vi "GxSingleCam.vi"() -> ()   [LabVIEW 2013]
uses:
  C:/Program Files/Daheng Imaging/GalaxySDK/Samples/LabVIEW SDK/x86/GxLVLib/dll/GxIAPINET.dll
  GxLVLib/dll/GxIAPINET.dll
  <vilib>/vision/Image Controls.llb/IMAQ Image.ctl
  GxLVLib/GxLVlib.lvlib
panel:
  out "是否退出":bool
  in  "图片存储路径":path
  in  "保存图片":bool
  in  "Image Src":T1
  out "Image":T1(plugin-control)
  out "采集回调":refnum<k27>
  out "是否支持白平衡":bool
  out "采集状态":bool
  out "设备状态":bool
  in  "IGxFactory":refnum<k24>
  in  "安全退出":bool
  in  "IGxStream":refnum<k24>
  in  "IGxDevice":refnum<k24>
  out "error out":errorcluster
  in  "发送软触发":bool
  in  "自动白平衡":string(combo)
  in  "增益":dbl format="%#_6f"
  in  "曝光时间":dbl
  in  "触发源":string(combo)
  in  "触发模式":string(combo)
  in  "停止采集":bool
  in  "开始采集":bool
  in  "关闭设备":bool
  in  "打开设备":bool
  # "触发模式"
  # "触发源"
  # "软触发"
  # "曝光时间(us)"
  # "增益(dB)"
  # "自动白平衡"
  # "保存图片"
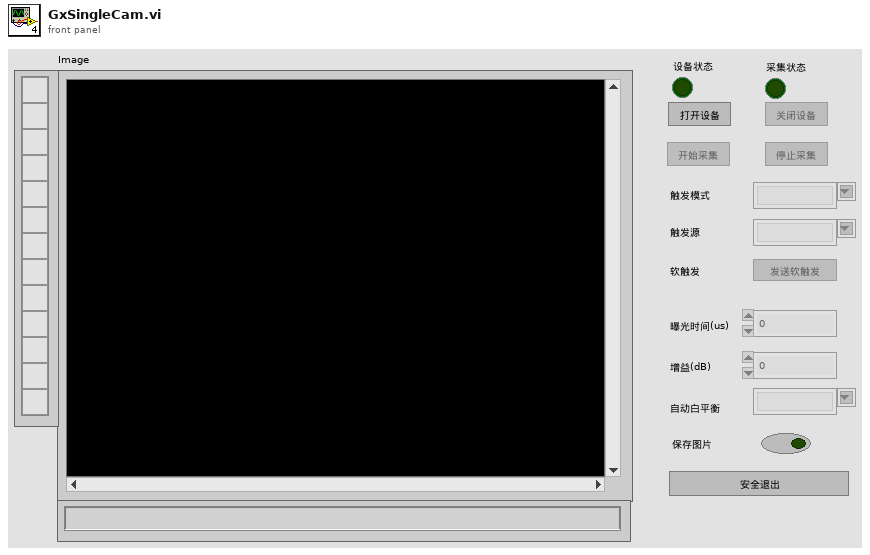
[diagram p1: front panel]
types:
  T1 = typedef "IMAQ Image.ctl" = refnum<image>
  T2 = typedef "Semaphore RefNum" = refnum<k1>
  T3 = enum8{"Enabled", "Disabled", "Disabled and Grayed Out"}
  T4 = typedef "Image Type" = u32
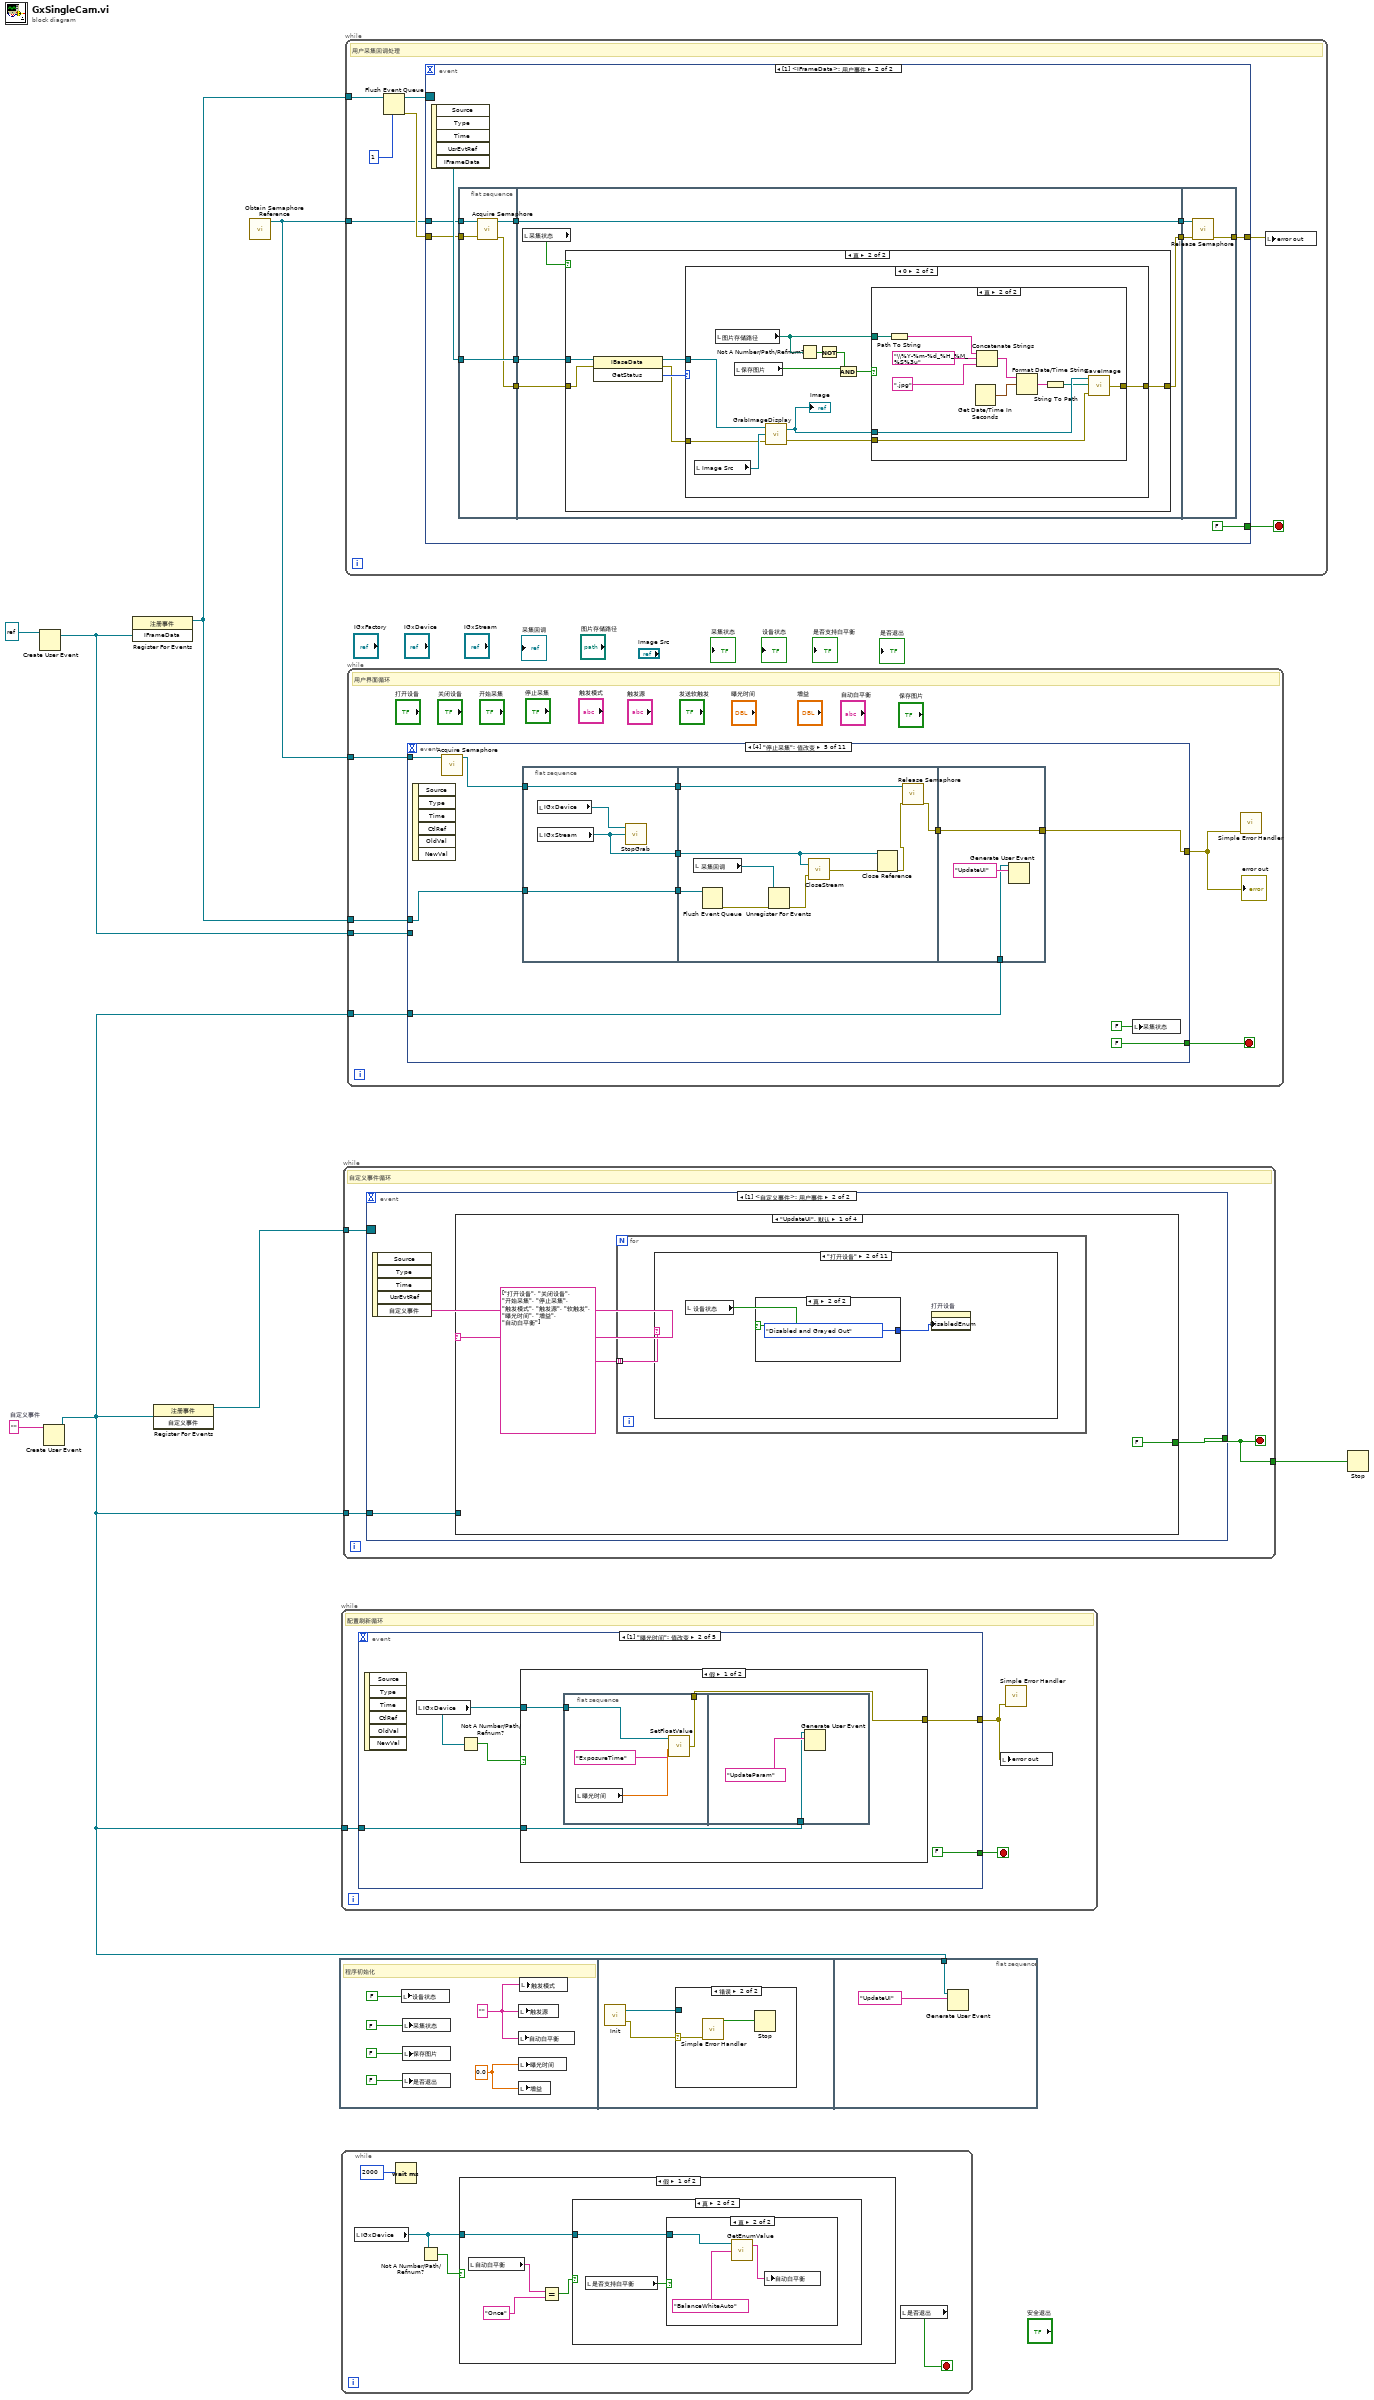
[diagram p0: block diagram]
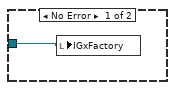
[diagram p5: hidden frame]
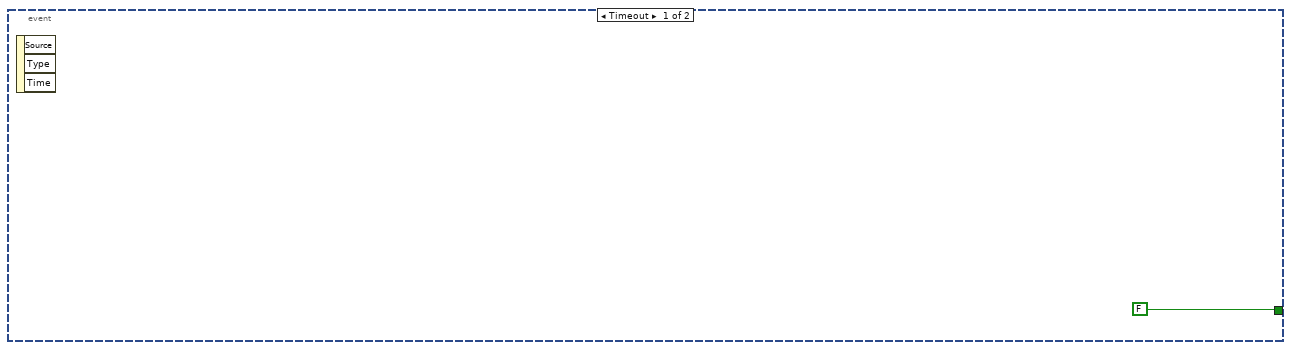
[diagram p6: hidden frame]
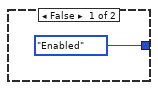
[diagram p8: hidden frame]
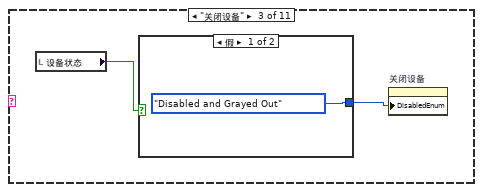
[diagram p9: hidden frame]
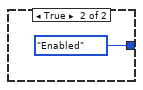
[diagram p10: hidden frame]
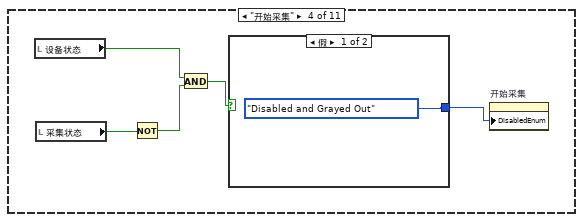
[diagram p11: hidden frame]
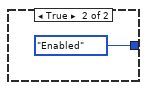
[diagram p12: hidden frame]
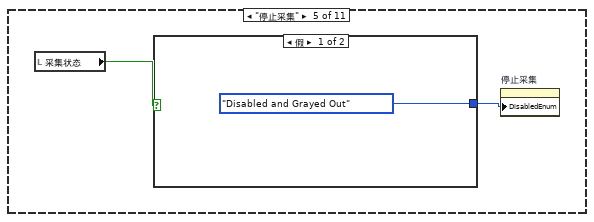
[diagram p13: hidden frame]
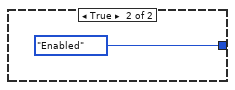
[diagram p14: hidden frame]
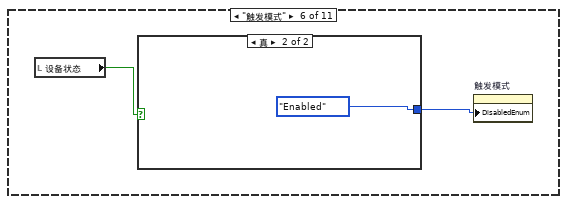
[diagram p15: hidden frame]
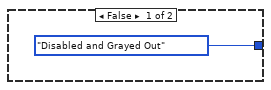
[diagram p16: hidden frame]
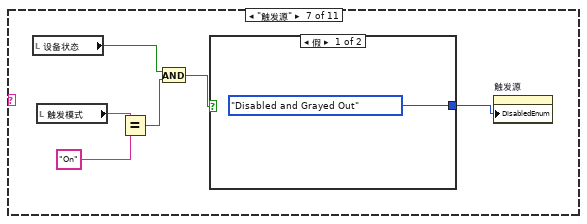
[diagram p17: hidden frame]
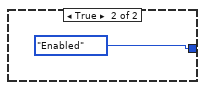
[diagram p18: hidden frame]
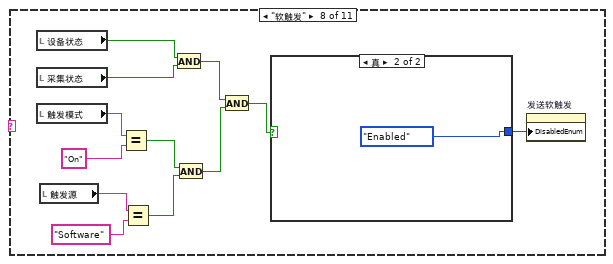
[diagram p19: hidden frame]
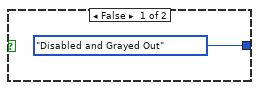
[diagram p20: hidden frame]
diagram:
  w6 = ""  # 自定义事件
  n1 = Create User Event(user event datatype=refnum<k24> refnum ("IFrameData")) -> (user event=w8:refnum<user-event>)  [unwired: 1 in, 1 out]
  n2 = Create User Event(user event datatype=w6) -> (user event=w3:refnum<user-event>)  [unwired: 1 in, 1 out]
  n3 = register-events(w8) -> (reference out=w2:refnum<event-registration>)  [unwired: 2 in, 1 out]
  n4 = register-events(w3) -> (reference out=w5:refnum<event-registration>)  [unwired: 2 in, 1 out]
  n5 = call <vilib>:"Obtain Semaphore Reference.vi"() -> ("semaphore"=w1:T2)  [unwired: 5 in, 2 out]
  n6 = flat-sequence {
    tunnel: w3 -> [w20]
    frame #0 {
      w11 = 0.0
      w12 = ""
      # "程序初始化"
      n7 = local write "设备状态"(FALSE) -> ()
      n8 = local write "采集状态"(FALSE) -> ()
      n9 = local write "保存图片"(FALSE) -> ()
      n10 = local write "是否退出"(FALSE) -> ()
      n11 = local write "自动白平衡"(w12) -> ()
      n12 = local write "触发源"(w12) -> ()
      n13 = local write "曝光时间"(w11) -> ()
      n14 = local write "增益"(w11) -> ()
      n15 = local write "触发模式"(w12) -> ()
    }
    frame #1 {
      n16 = call "Init.vi"() -> ("IGxFactory"=w16:refnum<k24>, "error out"=w15:errorcluster)  [unwired: 1 in]
      n17 = case shown="错误" w15 {
        selector: w15 -> [_ w18]
        tunnel: w16 -> [w17 _]
        frame No Error {
          n18 = local write "IGxFactory"(w17) -> ()
        }
        frame Error {
          n19 = call <vilib>:"Simple Error Handler.vi"("error in (no error)"=w18) -> ("error?"=w19:bool)  [unwired: 4 in, 4 out]
          n20 = Stop(stop? (T)=w19) -> ()
        }
      }
    }
    frame #2 {
      n21 = Generate User Event(user event=w20, event data cluster="UpdateUI") -> ()  [unwired: 2 in, 2 out]
    }
  }
  n22 = while {
    tunnel: w3 -> [w22]
    stop <- w24 stop-if-true
    # "配置刷新循环"
    n23 = event shown="[1] \"曝光时间\": 值改变" {
      selector: _ -> [_ _ _ _ _]
      dyn-events: _ -> [_ _ _ _ _]
      timeout: _ -> [_ _ _ _ _]
      tunnel: [errorcluster {FALSE, 0, ""} w29 w44 w59 errorcluster {"status"=FALSE, "code"=0, "source"=""} ("错误常量")] -> w23
      tunnel: [FALSE FALSE FALSE FALSE TRUE] -> w24
      tunnel: w22 -> [_ w27 w42 w57 _]
      event Timeout {
        n24 = event-data() -> ()  [unwired: 1 in, 3 out]
      }
      event "曝光时间": Value Change {
        n25 = event-data() -> ()  [unwired: 1 in, 6 out]
        n26 = local read "IGxDevice"() -> (w30:refnum<k24>)
        n27 = Not A Number/Path/Refnum?(number/path/refnum=w30) -> (NaN/Path/Refnum?=w31:bool)
        n28 = case shown="假" w31 {
          tunnel: w30 -> [w34 _]
          tunnel: [w33 errorcluster {TRUE, 5000, "GxSingleCam.vi"}] -> w29
          tunnel: w27 -> [w32 _]
          frame False {
            n29 = flat-sequence {
              tunnel: w34 -> [w36]
              tunnel: [w35] -> w33
              tunnel: w32 -> [w39]
              frame #0 {
                n30 = local read "曝光时间"() -> (w38:dbl)
                n31 = call "SetFloatValue.vi"("Float Value"=w38, "Feature Name"="ExposureTime", "IGxDevice"=w36) -> ("error out"=w35:errorcluster)  [unwired: 1 in]
              }
              frame #1 {
                n32 = Generate User Event(user event=w39, event data cluster="UpdateParam") -> ()  [unwired: 2 in, 2 out]
              }
            }
          }
          frame True {
          }
        }
      }
      event "增益": Value Change {
        n33 = event-data() -> ()  [unwired: 1 in, 6 out]
        n34 = local read "IGxDevice"() -> (w46:refnum<k24>)
        n35 = Not A Number/Path/Refnum?(number/path/refnum=w46) -> (NaN/Path/Refnum?=w45:bool)
        n36 = case shown="真" w45 {
          tunnel: w46 -> [w49 _]
          tunnel: [w48 errorcluster {TRUE, 0, "设备句柄无效"}] -> w44
          tunnel: w42 -> [w47 _]
          frame False {
            n37 = flat-sequence {
              tunnel: w49 -> [w51]
              tunnel: [w50] -> w48
              tunnel: w47 -> [w55]
              frame #0 {
                n38 = local read "增益"() -> (w53:dbl)
                n39 = call "SetFloatValue.vi"("Float Value"=w53, "Feature Name"="Gain", "IGxDevice"=w51) -> ("error out"=w50:errorcluster)  [unwired: 1 in]
              }
              frame #1 {
                n40 = Generate User Event(user event=w55, event data cluster="UpdateParam") -> ()  [unwired: 2 in, 2 out]
              }
            }
          }
          frame True {
          }
        }
      }
      event "自动白平衡": Value Change {
        n41 = event-data() -> ()  [unwired: 1 in, 6 out]
        n42 = local read "IGxDevice"() -> (w60:refnum<k24>)
        n43 = Not A Number/Path/Refnum?(number/path/refnum=w60) -> (NaN/Path/Refnum?=w61:bool)
        n44 = case shown="假" w61 {
          tunnel: w60 -> [w64 _]
          tunnel: [w63 errorcluster {TRUE, 0, "设备句柄无效"}] -> w59
          tunnel: w57 -> [w62 _]
          frame False {
            n45 = flat-sequence {
              tunnel: w64 -> [w66]
              tunnel: [w65] -> w63
              tunnel: w62 -> [w69]
              frame #0 {
                n46 = local read "自动白平衡"() -> (w68:string)
                n47 = call "SetEnumValue.vi"("Enum Value"=w68, "Feature Name"="BalanceWhiteAuto", "IGxDevice"=w66) -> ("error out"=w65:errorcluster)  [unwired: 1 in]
              }
              frame #1 {
                n48 = Generate User Event(user event=w69, event data cluster="UpdateParam") -> ()  [unwired: 2 in, 2 out]
              }
            }
          }
          frame True {
          }
        }
      }
      event "安全退出": Value Change {
        n49 = event-data() -> ()  [unwired: 1 in, 6 out]
      }
    }
    n50 = local write "error out"(w23) -> ()
    n51 = call <vilib>:"Simple Error Handler.vi"("error in (no error)"=w23) -> ()  [unwired: 4 in, 5 out]
  }
  n52 = while {
    stop <- w74 stop-if-true
    n53 = local read "IGxDevice"() -> (w76:refnum<k24>)
    n54 = Wait (ms)(milliseconds to wait=2000) -> ()  [unwired: 1 out]
    n55 = Not A Number/Path/Refnum?(number/path/refnum=w76) -> (NaN/Path/Refnum?=w75:bool)
    n56 = case shown="假" w75 {
      tunnel: w76 -> [w81 _]
      frame False {
        n57 = local read "自动白平衡"() -> (w79:string)
        n58 = Equal?(x=w79, y="Once") -> (x = y?=w78:bool)
        n59 = case shown="真" w78 {
          tunnel: w81 -> [_ w82]
          frame False {
          }
          frame True {
            n60 = local read "是否支持白平衡"() -> (w83:bool)
            n61 = case shown="真" w83 {
              tunnel: w82 -> [_ w86]
              frame False {
              }
              frame True {
                n62 = call "GetEnumValue.vi"("Feature Name"="BalanceWhiteAuto", "IGxDevice"=w86) -> ("Enum Value"=w84:string)  [unwired: 1 in, 1 out]
                n63 = local write "自动白平衡"(w84) -> ()
              }
            }
          }
        }
      }
      frame True {
      }
    }
    n64 = local read "是否退出"() -> (w74:bool)
  }
  n65 = while {
    tunnel: w5 -> [w89]
    tunnel: w3 -> [w88]
    tunnel: [w87] -> w4
    stop <- w87 stop-if-true
    # "自定义事件循环"
    n66 = event shown="[1] <自定义事件>: 用户事件" {
      selector: w89 -> [_ _]
      dyn-events: _ -> [_ _]
      timeout: _ -> [_ _]
      tunnel: [FALSE w91] -> w87
      tunnel: w88 -> [_ w92]
      event Timeout {
        n67 = event-data() -> ()  [unwired: 1 in, 3 out]
      }
      event User Event {
        n68 = event-data() -> ("自定义事件"=w93:string)  [unwired: 1 in, 4 out]
        n69 = case shown="\"UpdateUI\", 默认" w93 {
          tunnel: w92 -> [_ _ w224 _]
          tunnel: [FALSE TRUE FALSE FALSE] -> w91
          frame "UpdateUI", Default {
            n70 = for {
              tunnel: string[] ["打开设备", "关闭设备", "开始采集", "停止采集", "触发模式", "触发源", "软触发", "曝光时间", "增益", "自动白平衡"] -> [w96] mode=indexing
              n71 = case shown="\"打开设备\"" w96 {
                frame Default {
                }
                frame "打开设备" {
                  n72 = local read "设备状态"() -> (w98:bool)
                  n73 = case shown="真" w98 {
                    tunnel: [T3."Enabled" ("禁用") T3."Disabled and Grayed Out" ("禁用")] -> w97
                    frame False {
                    }
                    frame True {
                    }
                  }
                  n74 = property on="打开设备" class="Bool"("DisabledEnum"=w97) -> ()  [unwired: 2 in, 2 out]
                }
                frame "关闭设备" {
                  n75 = local read "设备状态"() -> (w102:bool)
                  n76 = case shown="假" w102 {
                    tunnel: [T3."Disabled and Grayed Out" ("禁用") T3."Enabled" ("禁用")] -> w101
                    frame False {
                    }
                    frame True {
                    }
                  }
                  n77 = property on="关闭设备" class="Bool"("DisabledEnum"=w101) -> ()  [unwired: 2 in, 2 out]
                }
                frame "开始采集" {
                  n78 = local read "设备状态"() -> (w108:bool)
                  n79 = local read "采集状态"() -> (w109:bool)
                  n80 = Not(x=w109) -> (.not. x?=w107:bool)
                  n81 = And(x=w108, y=w107) -> (x .and. y?=w106:bool)
                  n82 = case shown="假" w106 {
                    tunnel: [T3."Disabled and Grayed Out" ("禁用") T3."Enabled" ("禁用")] -> w105
                    frame False {
                    }
                    frame True {
                    }
                  }
                  n83 = property on="开始采集" class="Bool"("DisabledEnum"=w105) -> ()  [unwired: 2 in, 2 out]
                }
                frame "停止采集" {
                  n84 = local read "采集状态"() -> (w113:bool)
                  n85 = case shown="假" w113 {
                    tunnel: [T3."Disabled and Grayed Out" ("禁用") T3."Enabled" ("禁用")] -> w112
                    frame False {
                    }
                    frame True {
                    }
                  }
                  n86 = property on="停止采集" class="Bool"("DisabledEnum"=w112) -> ()  [unwired: 2 in, 2 out]
                }
                frame "触发模式" {
                  n87 = local read "设备状态"() -> (w117:bool)
                  n88 = case shown="真" w117 {
                    tunnel: [T3."Disabled and Grayed Out" ("禁用") T3."Enabled" ("禁用")] -> w116
                    frame False {
                    }
                    frame True {
                    }
                  }
                  n89 = property on="触发模式" class="CmbBox"("DisabledEnum"=w116) -> ()  [unwired: 2 in, 2 out]
                }
                frame "触发源" {
                  n90 = local read "设备状态"() -> (w123:bool)
                  n91 = local read "触发模式"() -> (w125:string)
                  n92 = Equal?(x=w125, y="On") -> (x = y?=w122:bool)
                  n93 = And(x=w123, y=w122) -> (x .and. y?=w121:bool)
                  n94 = case shown="假" w121 {
                    tunnel: [T3."Disabled and Grayed Out" ("禁用") T3."Enabled" ("禁用")] -> w120
                    frame False {
                    }
                    frame True {
                    }
                  }
                  n95 = property on="触发源" class="CmbBox"("DisabledEnum"=w120) -> ()  [unwired: 2 in, 2 out]
                }
                frame "软触发" {
                  n96 = local read "设备状态"() -> (w130:bool)
                  n97 = local read "采集状态"() -> (w129:bool)
                  n98 = local read "触发模式"() -> (w139:string)
                  n99 = local read "触发源"() -> (w137:string)
                  n100 = Equal?(x=w139, y="On") -> (x = y?=w135:bool)
                  n101 = Equal?(x=w137, y="Software") -> (x = y?=w134:bool)
                  n102 = And(x=w130, y=w129) -> (x .and. y?=w128:bool)
                  n103 = And(x=w135, y=w134) -> (x .and. y?=w133:bool)
                  n104 = And(x=w128, y=w133) -> (x .and. y?=w132:bool)
                  n105 = case shown="真" w132 {
                    tunnel: [T3."Disabled and Grayed Out" ("禁用") T3."Enabled" ("禁用")] -> w131
                    frame False {
                    }
                    frame True {
                    }
                  }
                  n106 = property on="发送软触发" class="Bool"("DisabledEnum"=w131) -> ()  [unwired: 2 in, 2 out]
                }
                frame "曝光时间" {
                  n107 = local read "设备状态"() -> (w143:bool)
                  n108 = case shown="假" w143 {
                    tunnel: [T3."Disabled and Grayed Out" ("禁用") T3."Enabled" ("禁用")] -> w142
                    frame False {
                    }
                    frame True {
                    }
                  }
                  n109 = property on="曝光时间" class="DigNum (严格)"("DisabledEnum"=w142) -> ()  [unwired: 2 in, 2 out]
                }
                frame "增益" {
                  n110 = local read "设备状态"() -> (w147:bool)
                  n111 = case shown="真" w147 {
                    tunnel: [T3."Disabled and Grayed Out" ("禁用") T3."Enabled" ("禁用")] -> w146
                    frame False {
                    }
                    frame True {
                    }
                  }
                  n112 = property on="增益" class="DigNum (严格)"("DisabledEnum"=w146) -> ()  [unwired: 2 in, 2 out]
                }
                frame "自动白平衡" {
                  n113 = local read "是否支持白平衡"() -> (w153:bool)
                  n114 = local read "设备状态"() -> (w152:bool)
                  n115 = And(x=w152, y=w153) -> (x .and. y?=w151:bool)
                  n116 = case shown="真" w151 {
                    tunnel: [T3."Disabled and Grayed Out" ("禁用") T3."Enabled" ("禁用")] -> w150
                    frame False {
                    }
                    frame True {
                    }
                  }
                  n117 = property on="自动白平衡" class="CmbBox"("DisabledEnum"=w150) -> ()  [unwired: 2 in, 2 out]
                }
              }
            }
          }
          frame "Quit" {
            n118 = for {
              tunnel: string[] ["打开设备", "关闭设备", "开始采集", "停止采集", "触发模式", "触发源", "软触发", "曝光时间", "增益", "自动白平衡"] -> [w160] mode=indexing
              n119 = case shown="\"停止采集\"" w160 {
                frame Default {
                }
                frame "打开设备" {
                  n120 = local read "设备状态"() -> (w162:bool)
                  n121 = case shown="真" w162 {
                    tunnel: [T3."Enabled" ("禁用") T3."Disabled and Grayed Out" ("禁用")] -> w161
                    frame False {
                    }
                    frame True {
                    }
                  }
                  n122 = property on="打开设备" class="Bool"("DisabledEnum"=w161) -> ()  [unwired: 2 in, 2 out]
                }
                frame "关闭设备" {
                  n123 = local read "设备状态"() -> (w166:bool)
                  n124 = case shown="假" w166 {
                    tunnel: [T3."Disabled and Grayed Out" ("禁用") T3."Enabled" ("禁用")] -> w165
                    frame False {
                    }
                    frame True {
                    }
                  }
                  n125 = property on="关闭设备" class="Bool"("DisabledEnum"=w165) -> ()  [unwired: 2 in, 2 out]
                }
                frame "开始采集" {
                  n126 = local read "设备状态"() -> (w172:bool)
                  n127 = local read "采集状态"() -> (w173:bool)
                  n128 = Not(x=w173) -> (.not. x?=w171:bool)
                  n129 = And(x=w172, y=w171) -> (x .and. y?=w170:bool)
                  n130 = case shown="假" w170 {
                    tunnel: [T3."Disabled and Grayed Out" ("禁用") T3."Enabled" ("禁用")] -> w169
                    frame False {
                    }
                    frame True {
                    }
                  }
                  n131 = property on="开始采集" class="Bool"("DisabledEnum"=w169) -> ()  [unwired: 2 in, 2 out]
                }
                frame "停止采集" {
                  n132 = local read "采集状态"() -> (w177:bool)
                  n133 = case shown="假" w177 {
                    tunnel: [T3."Disabled and Grayed Out" ("禁用") T3."Enabled" ("禁用")] -> w176
                    frame False {
                    }
                    frame True {
                    }
                  }
                  n134 = property on="停止采集" class="Bool"("DisabledEnum"=w176) -> ()  [unwired: 2 in, 2 out]
                }
                frame "触发模式" {
                  n135 = local read "设备状态"() -> (w181:bool)
                  n136 = case shown="真" w181 {
                    tunnel: [T3."Disabled and Grayed Out" ("禁用") T3."Enabled" ("禁用")] -> w180
                    frame False {
                    }
                    frame True {
                    }
                  }
                  n137 = property on="触发模式" class="CmbBox"("DisabledEnum"=w180) -> ()  [unwired: 2 in, 2 out]
                }
                frame "触发源" {
                  n138 = local read "设备状态"() -> (w187:bool)
                  n139 = local read "触发模式"() -> (w189:string)
                  n140 = Equal?(x=w189, y="On") -> (x = y?=w186:bool)
                  n141 = And(x=w187, y=w186) -> (x .and. y?=w185:bool)
                  n142 = case shown="假" w185 {
                    tunnel: [T3."Disabled and Grayed Out" ("禁用") T3."Enabled" ("禁用")] -> w184
                    frame False {
                    }
                    frame True {
                    }
                  }
                  n143 = property on="触发源" class="CmbBox"("DisabledEnum"=w184) -> ()  [unwired: 2 in, 2 out]
                }
                frame "软触发" {
                  n144 = local read "设备状态"() -> (w194:bool)
                  n145 = local read "采集状态"() -> (w193:bool)
                  n146 = local read "触发模式"() -> (w203:string)
                  n147 = local read "触发源"() -> (w201:string)
                  n148 = Equal?(x=w203, y="On") -> (x = y?=w199:bool)
                  n149 = Equal?(x=w201, y="Software") -> (x = y?=w198:bool)
                  n150 = And(x=w194, y=w193) -> (x .and. y?=w192:bool)
                  n151 = And(x=w199, y=w198) -> (x .and. y?=w197:bool)
                  n152 = And(x=w192, y=w197) -> (x .and. y?=w196:bool)
                  n153 = case shown="真" w196 {
                    tunnel: [T3."Disabled and Grayed Out" ("禁用") T3."Enabled" ("禁用")] -> w195
                    frame False {
                    }
                    frame True {
                    }
                  }
                  n154 = property on="发送软触发" class="Bool"("DisabledEnum"=w195) -> ()  [unwired: 2 in, 2 out]
                }
                frame "曝光时间" {
                  n155 = local read "设备状态"() -> (w207:bool)
                  n156 = case shown="假" w207 {
                    tunnel: [T3."Disabled and Grayed Out" ("禁用") T3."Enabled" ("禁用")] -> w206
                    frame False {
                    }
                    frame True {
                    }
                  }
                  n157 = property on="曝光时间" class="DigNum (严格)"("DisabledEnum"=w206) -> ()  [unwired: 2 in, 2 out]
                }
                frame "增益" {
                  n158 = local read "设备状态"() -> (w211:bool)
                  n159 = case shown="真" w211 {
                    tunnel: [T3."Disabled and Grayed Out" ("禁用") T3."Enabled" ("禁用")] -> w210
                    frame False {
                    }
                    frame True {
                    }
                  }
                  n160 = property on="增益" class="DigNum (严格)"("DisabledEnum"=w210) -> ()  [unwired: 2 in, 2 out]
                }
                frame "自动白平衡" {
                  n161 = local read "是否支持白平衡"() -> (w217:bool)
                  n162 = local read "设备状态"() -> (w216:bool)
                  n163 = And(x=w216, y=w217) -> (x .and. y?=w215:bool)
                  n164 = case shown="真" w215 {
                    tunnel: [T3."Disabled and Grayed Out" ("禁用") T3."Enabled" ("禁用")] -> w214
                    frame False {
                    }
                    frame True {
                    }
                  }
                  n165 = property on="自动白平衡" class="CmbBox"("DisabledEnum"=w214) -> ()  [unwired: 2 in, 2 out]
                }
              }
            }
            n166 = local read "IGxFactory"() -> (w156:refnum<k24>)
            n167 = call "UnInit.vi"("IGxFactory"=w156) -> ("error out"=w157:errorcluster)  [unwired: 1 in]
            n168 = Close Reference(reference=w156, error in (no error)=w157) -> ()  [unwired: 1 out]
          }
          frame "UpdateParam" {
            n169 = local read "IGxDevice"() -> (w226:refnum<k24>)
            n170 = local read "设备状态"() -> (w230:bool)
            n171 = Not A Number/Path/Refnum?(number/path/refnum=w226) -> (NaN/Path/Refnum?=w227:bool)
            n172 = Not(x=w227) -> (.not. x?=w229:bool)
            n173 = And(x=w229, y=w230) -> (x .and. y?=w228:bool)
            n174 = case shown="真" w228 {
              tunnel: [errorcluster {FALSE, 0, ""} w232] -> w223
              tunnel: string[] ["TriggerMode", "TriggerSource", "ExposureTime", "Gain", "BalanceWhiteAuto"] -> [_ w235]
              tunnel: w226 -> [_ w234]
              frame False {
              }
              frame True {
                n175 = for {
                  tunnel: w235 -> [w238] mode=indexing
                  tunnel: w234 -> [w237]
                  tunnel: [w236] -> w233 mode=indexing
                  n176 = case shown="\"BalanceWhiteAuto\"" w238 {
                    selector: w238 -> [w241 w245 w249 w253 w256]
                    tunnel: w237 -> [w242 w246 w250 w254 w257]
                    tunnel: [w239 w243 w247 w251 w259] -> w236
                    frame "TriggerMode", Default {
                      n177 = call "GetEnumValue.vi"("Feature Name"=w241, "IGxDevice"=w242) -> ("error out"=w239:errorcluster, "Enum Value"=w240:string)  [unwired: 1 in]
                      n178 = local write "触发模式"(w240) -> ()
                    }
                    frame "TriggerSource" {
                      n179 = call "GetEnumValue.vi"("Feature Name"=w245, "IGxDevice"=w246) -> ("error out"=w243:errorcluster, "Enum Value"=w244:string)  [unwired: 1 in]
                      n180 = local write "触发源"(w244) -> ()
                    }
                    frame "ExposureTime" {
                      n181 = call "GetFloatValue.vi"("Feature Name"=w249, "IGxDevice"=w250) -> ("error out"=w247:errorcluster, "Float Value"=w248:dbl)  [unwired: 1 in]
                      n182 = local write "曝光时间"(w248) -> ()
                    }
                    frame "Gain" {
                      n183 = call "GetFloatValue.vi"("Feature Name"=w253, "IGxDevice"=w254) -> ("error out"=w251:errorcluster, "Float Value"=w252:dbl)  [unwired: 1 in]
                      n184 = local write "增益"(w252) -> ()
                    }
                    frame "BalanceWhiteAuto" {
                      n185 = call "IsImplemented.vi"("Feature Name"=w256, "IGxDevice"=w257) -> ("error out"=w258:errorcluster, "IsImplement"=w255:bool)  [unwired: 1 in]
                      n186 = local write "是否支持白平衡"(w255) -> ()
                      n187 = case shown="真" w255 {
                        tunnel: [w260 w264] -> w259
                        tunnel: w258 -> [w260 w265]
                        tunnel: w257 -> [_ w262]
                        tunnel: w256 -> [_ w261]
                        frame False {
                        }
                        frame True {
                          n188 = call "GetEnumValue.vi"("error in (no error)"=w265, "Feature Name"=w261, "IGxDevice"=w262) -> ("error out"=w264:errorcluster, "Enum Value"=w263:string)
                          n189 = local write "自动白平衡"(w263) -> ()
                        }
                      }
                    }
                  }
                }
                n190 = Merge Errors(w233) -> (w232:errorcluster)
              }
            }
            n191 = Generate User Event(user event=w224, event data cluster="UpdateUI", error in=w223) -> (error out=w222:errorcluster)  [unwired: 1 in, 1 out]
            n192 = local write "error out"(w222) -> ()
            n193 = call <vilib>:"Simple Error Handler.vi"("error in (no error)"=w222) -> ()  [unwired: 4 in, 5 out]
          }
          frame "PicShow" {
            n194 = local read "IGxDevice"() -> (w268:refnum<k24>)
            n195 = local read "设备状态"() -> (w272:bool)
            n196 = Not A Number/Path/Refnum?(number/path/refnum=w268) -> (NaN/Path/Refnum?=w269:bool)
            n197 = Not(x=w269) -> (.not. x?=w271:bool)
            n198 = And(x=w271, y=w272) -> (x .and. y?=w270:bool)
            n199 = case shown="真" w270 {
              tunnel: [errorcluster {FALSE, 0, ""} errorcluster {FALSE, 0, ""}] -> w266
              tunnel: w268 -> [_ w278]
              frame False {
              }
              frame True {
                n200 = call "IsImplemented.vi"("Feature Name"="PixelColorFilter", "IGxDevice"=w278) -> ("IsImplement"=w280:bool)  [unwired: 1 in, 1 out]
                n201 = case shown="真" w280 {
                  tunnel: w278 -> [_ w287]
                  tunnel: [w281 w282] -> w275
                  frame False {
                    w281 = T4 0 items=["Grayscale (U8)", "Grayscale (I16)", "Grayscale (SGL)", "Complex (CSG)", "RGB (U32)", "HSL (U32)", "RGB (U64)", "Grayscale (U16)"] ("Image Type")
                  }
                  frame True {
                    n202 = call "GetEnumValue.vi"("Feature Name"="PixelColorFilter", "IGxDevice"=w287) -> ("Enum Value"=w285:string)  [unwired: 1 in, 1 out]
                    n203 = Equal?(x=w285, y="None") -> (x = y?=w283:bool)
                    n204 = case shown="假" w283 {
                      tunnel: [w288 w289] -> w282
                      frame False {
                        w288 = T4 4 items=["Grayscale (U8)", "Grayscale (I16)", "Grayscale (SGL)", "Complex (CSG)", "RGB (U32)", "HSL (U32)", "RGB (U64)", "Grayscale (U16)"] ("Image Type")
                      }
                      frame True {
                        w289 = T4 0 items=["Grayscale (U8)", "Grayscale (I16)", "Grayscale (SGL)", "Complex (CSG)", "RGB (U32)", "HSL (U32)", "RGB (U64)", "Grayscale (U16)"] ("Image Type")
                      }
                    }
                  }
                }
                n205 = call "IMAQ Create"("Image Name"="", "Image Type"=w275) -> ("New Image"=w276:T1)  [unwired: 3 in, 1 out]
                n206 = local write "Image Src"(w276) -> ()
              }
            }
            n207 = local write "error out"(w266) -> ()
            n208 = call <vilib>:"Simple Error Handler.vi"("error in (no error)"=w266) -> ()  [unwired: 4 in, 5 out]
          }
        }
      }
    }
  }
  n209 = while {
    tunnel: w2 -> [w295]
    tunnel: w1 -> [w290]
    stop <- w296 stop-if-true
    # "用户采集回调处理"
    n210 = Flush Event Queue(0:w295, 5:1) -> (8:w294:refnum<event-registration>, 11:w291:errorcluster)  [unwired: 4 in, 1 out]
    n211 = event shown="[1] <IFrameData>: 用户事件" {
      selector: w294 -> [_ _]
      dyn-events: _ -> [_ _]
      timeout: _ -> [_ _]
      tunnel: [_ FALSE] -> w296
      tunnel: [w297 w298] -> w292
      tunnel: w291 -> [w297 w301]
      tunnel: w290 -> [_ w304]
      event Timeout {
        n212 = event-data() -> ()  [unwired: 1 in, 3 out]
      }
      event User Event {
        n213 = event-data() -> ("IFrameData"=w306:refnum<k24>)  [unwired: 1 in, 4 out]
        n214 = flat-sequence {
          tunnel: w306 -> [w312]
          tunnel: [w312] -> w305
          tunnel: w304 -> [w311]
          tunnel: [w310] -> w302
          tunnel: w301 -> [w309]
          tunnel: [w308] -> w300
          tunnel: w305 -> [w317]
          tunnel: [w316] -> w303
          tunnel: w302 -> [w316]
          tunnel: w300 -> [w315]
          tunnel: [w314] -> w299
          tunnel: w303 -> [w351]
          tunnel: w299 -> [w350]
          tunnel: [w349] -> w298
          frame #0 {
            n215 = call <vilib>:"Acquire Semaphore.vi"("error in (no error)"=w309, "semaphore"=w311) -> ("error out"=w308:errorcluster, "semaphore out"=w310:T2)  [unwired: 3 in, 1 out]
          }
          frame #1 {
            n216 = local read "采集状态"() -> (w313:bool)
            n217 = case shown="真" w313 {
              tunnel: [w318 w321] -> w314
              tunnel: w317 -> [_ w320]
              tunnel: w315 -> [w318 w319]
              frame False {
              }
              frame True {
                n218 = invoke class="IBaseData" method="GetStatus"(reference=w320, error in=w319) -> (reference out=w323:refnum<k24>, error out=w322:errorcluster, "GetStatus"=w324:i32)  [unwired: 1 in]
                n219 = case shown="0" w324 {
                  tunnel: [w325 w330] -> w321
                  tunnel: w323 -> [_ w326]
                  tunnel: w322 -> [w325 w327]
                  frame Default {
                  }
                  frame 0 {
                    n220 = local read "Image Src"() -> (w331:T1)
                    n221 = local read "图片存储路径"() -> (w329:path)
                    n222 = local read "保存图片"() -> (w334:bool)
                    n223 = call "GrabImageDisplay.vi"("error in (no error)"=w327, "Image Src"=w331, "IBaseData"=w326) -> ("error out"=w336:errorcluster, "Image out"=w328:T1)
                    "Image" <- w328
                    n224 = Not A Number/Path/Refnum?(number/path/refnum=w329) -> (NaN/Path/Refnum?=w332:bool)
                    n225 = Not(x=w332) -> (.not. x?=w333:bool)
                    n226 = And(x=w334, y=w333) -> (x .and. y?=w335:bool)
                    n227 = case shown="真" w335 {
                      tunnel: w329 -> [_ w344]
                      tunnel: w328 -> [_ w343]
                      tunnel: w336 -> [w337 w341]
                      tunnel: [w337 w340] -> w330
                      frame False {
                      }
                      frame True {
                        n228 = Path To String(path=w344) -> (string=w345:string)
                        n229 = Get Date/Time In Seconds() -> (seconds since 1Jan1904=w347:timestamp)
                        n230 = Concatenate Strings(w345, "\\%Y-%m-%d_%H_%M_%S%3u", ".jpg") -> (w346:string)
                        n231 = Format Date/Time String(time format string (%c)=w346, seconds (now)=w347) -> (date/time string=w348:string)  [unwired: 1 in]
                        n232 = String To Path(string=w348) -> (path=w342:path)
                        n233 = call "SaveImage.vi"("error in (no error)"=w341, "Path"=w342, "Image Src"=w343) -> ("error out"=w340:errorcluster)
                      }
                    }
                  }
                }
              }
            }
          }
          frame #2 {
            n234 = call <vilib>:"Release Semaphore.vi"("error in (no error)"=w350, "semaphore"=w351) -> ("error out"=w349:errorcluster)  [unwired: 4 in, 1 out]
          }
        }
      }
    }
    n235 = local write "error out"(w292) -> ()
  }
  n236 = while {
    tunnel: w8 -> [w357]
    tunnel: w3 -> [w356]
    tunnel: w2 -> [w353]
    tunnel: w1 -> [w352]
    stop <- w354 stop-if-true
    # "用户界面循环"
    n237 = event shown="[4] \"停止采集\": 值改变" {
      selector: _ -> [_ _ _ _ _ _ _ _ _ _ _]
      dyn-events: _ -> [_ _ _ _ _ _ _ _ _ _ _]
      timeout: _ -> [_ _ _ _ _ _ _ _ _ _ _]
      tunnel: [errorcluster {FALSE, 0, ""} w362 _ w432 w462 w490 w498 w505 _ _ _] -> w355
      tunnel: [FALSE FALSE FALSE FALSE FALSE FALSE FALSE FALSE FALSE TRUE TRUE] -> w354
      tunnel: w357 -> [_ _ _ w433 _ _ _ _ _ _ _]
      tunnel: w356 -> [_ w360 w391 w430 w463 w492 w499 w507 _ w525 w567]
      tunnel: w353 -> [_ _ w390 _ w464 _ _ _ _ w526 w568]
      tunnel: w352 -> [_ _ w389 _ w471 _ _ _ _ w524 w566]
      event Timeout {
        n238 = event-data() -> ()  [unwired: 1 in, 3 out]
      }
      event "打开设备": Value Change {
        n239 = event-data() -> ()  [unwired: 1 in, 6 out]
        n240 = flat-sequence {
          tunnel: [w366] -> w361
          tunnel: [w388] -> w362
          tunnel: w361 -> [w388]
          tunnel: w360 -> [w385]
          frame #0 {
            n241 = local read "IGxFactory"() -> (w367:refnum<k24>)
            n242 = call "UpdateDeviceList.vi"("time out"=1000, "IGxFactory"=w367) -> ("error out"=w364:errorcluster, "DeviceSNList"=w365:string[])  [unwired: 1 in]
            n243 = Array Size(array=w365) -> (size(s)=w368:i32)
            n244 = case shown="默认" w368 {
              tunnel: w365 -> [w377 _]
              tunnel: w367 -> [w373 _]
              tunnel: [w372 w383] -> w366
              tunnel: w364 -> [w371 w384]
              frame Default {
                n245 = Index Array(array=w377, index=0) -> (element=w374:string)
                n246 = call "OpenDeviceBySN.vi"("error in (no error)"=w371, "SN"=w374, "IGxFactory"=w373) -> ("error out"=w370:errorcluster, "IGxDevice"=w375:refnum<k24>)
                n247 = case shown="无错误" w370 {
                  selector: w370 -> [w378 w381]
                  tunnel: w375 -> [w379 _]
                  tunnel: [w378 w381] -> w372
                  frame No Error {
                    n248 = local write "IGxDevice"(w379) -> ()
                    n249 = local write "设备状态"(TRUE) -> ()
                  }
                  frame Error {
                  }
                }
              }
              frame 0 {
                n250 = Merge Errors(w384, errorcluster {TRUE, 5001, "GxSingleCam.vi"}) -> (w383:errorcluster)
              }
            }
          }
          frame #1 {
            n251 = Generate User Event(user event=w385, event data cluster="UpdateParam") -> ()  [unwired: 2 in, 2 out]
            n252 = Generate User Event(user event=w385, event data cluster="PicShow") -> ()  [unwired: 2 in, 2 out]
          }
        }
      }
      event "关闭设备": Value Change {
        n253 = event-data() -> ()  [unwired: 1 in, 6 out]
        n254 = flat-sequence {
          tunnel: w390 -> [w396]
          tunnel: w389 -> [w395]
          tunnel: w391 -> [w428]
          frame #0 {
            n255 = local read "IGxStream"() -> (w400:refnum<k24>)
            n256 = local read "IGxDevice"() -> (w399:refnum<k24>)
            n257 = Not A Number/Path/Refnum?(number/path/refnum=w400) -> (NaN/Path/Refnum?=w401:bool)
            n258 = case shown="假" w401 {
              tunnel: w400 -> [w414 _]
              tunnel: w399 -> [w412 w427]
              tunnel: w396 -> [w409 _]
              tunnel: [w411 w427] -> w397
              tunnel: w395 -> [w407 _]
              frame False {
                n259 = call <vilib>:"Acquire Semaphore.vi"("semaphore"=w407) -> ("semaphore out"=w406:T2)  [unwired: 4 in, 2 out]
                n260 = flat-sequence {
                  tunnel: w414 -> [w417]
                  tunnel: [w418] -> w413
                  tunnel: w412 -> [w418]
                  tunnel: [w416] -> w410
                  tunnel: w409 -> [w416]
                  tunnel: [w417] -> w408
                  tunnel: w406 -> [w415]
                  tunnel: [w415] -> w405
                  tunnel: w413 -> [w426]
                  tunnel: [w426] -> w411
                  tunnel: w410 -> [w425]
                  tunnel: w408 -> [w421]
                  tunnel: [w419] -> w404
                  tunnel: w405 -> [w419]
                  frame #0 {
                    n261 = call "StopGrab.vi"("IGxStream"=w417, "IGxDevice"=w418) -> ()  [unwired: 1 in, 1 out]
                  }
                  frame #1 {
                    n262 = local read "采集回调"() -> (w423:refnum<k27>)
                    n263 = Flush Event Queue(0:w425) -> (11:w424:errorcluster)  [unwired: 5 in, 2 out]
                    n264 = Unregister For Events(event registration refnum=w423, error in=w424) -> (error out=w420:errorcluster)
                    n265 = call "CloseStream.vi"("error in (no error)"=w420, "IGxStream"=w421) -> ("error out"=w422:errorcluster)
                    n266 = Close Reference(reference=w421, error in (no error)=w422) -> ()  [unwired: 1 out]
                  }
                }
                n267 = call <vilib>:"Release Semaphore.vi"("semaphore"=w404) -> ()  [unwired: 5 in, 2 out]
              }
              frame True {
              }
            }
            n268 = local read "Image Src"() -> (w402:T1)
            n269 = call "CloseDevice.vi"("IGxDevice"=w397) -> ("error out"=w403:errorcluster)  [unwired: 1 in]
            n270 = Close Reference(reference=w397, error in (no error)=w403) -> (error out=w398:errorcluster)
            n271 = call "Imaq Dispose"("Image"=w402, "error in (no error)"=w398) -> ()  [unwired: 1 in, 4 out]
          }
          frame #1 {
            n272 = Generate User Event(user event=w428, event data cluster="UpdateUI") -> ()  [unwired: 2 in, 2 out]
          }
        }
        n273 = local write "采集状态"(FALSE) -> ()
        n274 = local write "设备状态"(FALSE) -> ()
      }
      event "开始采集": Value Change {
        n275 = event-data() -> ()  [unwired: 1 in, 6 out]
        n276 = flat-sequence {
          tunnel: w433 -> [w442]
          tunnel: [w436] -> w431
          tunnel: [w461] -> w432
          tunnel: w431 -> [w461]
          tunnel: w430 -> [w459]
          frame #0 {
            n277 = local read "IGxDevice"() -> (w444:refnum<k24>)
            n278 = vi-ref "ImageGrabEvent.vi"() -> (w437:refnum<vi>)
            n279 = call "OpenStream.vi"("StreamID"=0, "IGxDevice"=w444) -> ("error out"=w441:errorcluster, "IGxStream"=w439:refnum<k24>)  [unwired: 1 in]
            n280 = node(w441, w439, w437, w442) -> (w438:refnum<k27>, w440:errorcluster)  [unwired: 1 in]
            n281 = local write "采集回调"(w438) -> ()
            n282 = local write "IGxStream"(w439) -> ()
            n283 = call "StartGrab.vi"("error in (no error)"=w440, "IGxStream"=w439, "IGxDevice"=w444) -> ("error out"=w435:errorcluster)
            n284 = case shown="错误" w435 {
              selector: w435 -> [w445 w448]
              tunnel: w439 -> [_ w452]
              tunnel: w438 -> [_ w453]
              tunnel: [w445 w449] -> w436
              frame No Error {
                n285 = local write "采集状态"(TRUE) -> ()
              }
              frame Error {
                n286 = Not A Number/Path/Refnum?(number/path/refnum=w453) -> (NaN/Path/Refnum?=w454:bool)
                n287 = call "CloseStream.vi"("IGxStream"=w452) -> ("error out"=w451:errorcluster)  [unwired: 1 in]
                n288 = Close Reference(reference=w452, error in (no error)=w451) -> (error out=w450:errorcluster)
                n289 = case shown="假" w454 {
                  tunnel: w453 -> [w457 _]
                  tunnel: [w456 w458] -> w447
                  tunnel: w450 -> [w455 w458]
                  frame False {
                    n290 = Unregister For Events(event registration refnum=w457, error in=w455) -> (error out=w456:errorcluster)
                  }
                  frame True {
                  }
                }
                n291 = Merge Errors(w448, w447) -> (w449:errorcluster)
              }
            }
          }
          frame #1 {
            n292 = Generate User Event(user event=w459, event data cluster="UpdateUI") -> ()  [unwired: 2 in, 2 out]
          }
        }
      }
      event "停止采集": Value Change {
        n293 = event-data() -> ()  [unwired: 1 in, 6 out]
        n294 = call <vilib>:"Acquire Semaphore.vi"("semaphore"=w471) -> ("semaphore out"=w466:T2)  [unwired: 4 in, 2 out]
        n295 = flat-sequence {
          tunnel: [w473] -> w469
          tunnel: [w475] -> w468
          tunnel: w466 -> [w474]
          tunnel: [w474] -> w465
          tunnel: w464 -> [w473]
          tunnel: [w478] -> w467
          tunnel: w469 -> [w485]
          tunnel: w468 -> [w481]
          tunnel: w465 -> [w477]
          tunnel: [w488] -> w462
          tunnel: w467 -> [w488]
          tunnel: w463 -> [w486]
          frame #0 {
            n296 = local read "IGxDevice"() -> (w476:refnum<k24>)
            n297 = local read "IGxStream"() -> (w475:refnum<k24>)
            n298 = call "StopGrab.vi"("IGxStream"=w475, "IGxDevice"=w476) -> ()  [unwired: 1 in, 1 out]
          }
          frame #1 {
            n299 = local read "采集回调"() -> (w484:refnum<k27>)
            n300 = Flush Event Queue(0:w485) -> (11:w483:errorcluster)  [unwired: 5 in, 2 out]
            n301 = Unregister For Events(event registration refnum=w484, error in=w483) -> (error out=w480:errorcluster)
            n302 = call "CloseStream.vi"("error in (no error)"=w480, "IGxStream"=w481) -> ("error out"=w482:errorcluster)
            n303 = Close Reference(reference=w481, error in (no error)=w482) -> (error out=w479:errorcluster)
            n304 = call <vilib>:"Release Semaphore.vi"("error in (no error)"=w479, "semaphore"=w477) -> ("error out"=w478:errorcluster)  [unwired: 4 in, 1 out]
          }
          frame #2 {
            n305 = Generate User Event(user event=w486, event data cluster="UpdateUI") -> ()  [unwired: 2 in, 2 out]
          }
        }
        n306 = local write "采集状态"(FALSE) -> ()
      }
      event "触发模式": Value Change {
        n307 = event-data() -> ()  [unwired: 1 in, 6 out]
        n308 = local read "IGxDevice"() -> (w496:refnum<k24>)
        n309 = local read "触发模式"() -> (w495:string)
        n310 = call "SetEnumValue.vi"("Enum Value"=w495, "Feature Name"="TriggerMode", "IGxDevice"=w496) -> ("error out"=w491:errorcluster)  [unwired: 1 in]
        n311 = Generate User Event(user event=w492, event data cluster="UpdateParam", error in=w491) -> (error out=w490:errorcluster)  [unwired: 1 in, 1 out]
      }
      event "触发源": Value Change {
        n312 = event-data() -> ()  [unwired: 1 in, 6 out]
        n313 = local read "IGxDevice"() -> (w504:refnum<k24>)
        n314 = local read "触发源"() -> (w502:string)
        n315 = call "SetEnumValue.vi"("Enum Value"=w502, "Feature Name"="TriggerSource", "IGxDevice"=w504) -> ("error out"=w500:errorcluster)  [unwired: 1 in]
        n316 = Generate User Event(user event=w499, event data cluster="UpdateUI", error in=w500) -> (error out=w498:errorcluster)  [unwired: 1 in, 1 out]
      }
      event "发送软触发": Value Change {
        n317 = event-data() -> ()  [unwired: 1 in, 6 out]
        n318 = local read "IGxDevice"() -> (w511:refnum<k24>)
        n319 = call "SetCommandValue.vi"("Feature Name"="TriggerSoftware", "IGxDevice"=w511) -> ("error out"=w508:errorcluster)  [unwired: 1 in]
        n320 = Generate User Event(user event=w507, event data cluster="UpdateUI", error in=w508) -> (error out=w505:errorcluster)  [unwired: 1 in, 1 out]
      }
      event "保存图片": Value Change {
        n321 = event-data() -> ()  [unwired: 1 in, 6 out]
        n322 = local read "保存图片"() -> (w513:bool)
        n323 = case shown="真" w513 {
          frame False {
          }
          frame True {
            n324 = call <vilib>:"Application Directory.vi"() -> ("Application Directory"=w520:path)
            n325 = Path To String(path=w520) -> (string=w519:string)
            n326 = Concatenate Strings(w519, "\\Image") -> (w517:string)
            n327 = String To Path(string=w517) -> (path=w515:path)
            n328 = call <vilib>:"Check if File or Folder Exists.vi"("path"=w515) -> ("file or folder exists?"=w516:bool)  [unwired: 8 in, 2 out]
            n329 = case shown="假" w516 {
              tunnel: w515 -> [w522 w523]
              tunnel: [w521 w523] -> w514
              frame False {
                n330 = Create Folder(path (use dialog)=w522) -> (created path=w521:path)  [unwired: 2 in, 2 out]
              }
              frame True {
              }
            }
            n331 = local write "图片存储路径"(w514) -> ()
          }
        }
      }
      event "安全退出": Value Change {
        n332 = event-data() -> ()  [unwired: 1 in, 6 out]
        n333 = flat-sequence {
          tunnel: w526 -> [w531]
          tunnel: w524 -> [w528]
          tunnel: w525 -> [w564]
          frame #0 {
            n334 = local read "采集状态"() -> (w532:bool)
            n335 = local read "IGxDevice"() -> (w530:refnum<k24>)
            n336 = local read "IGxStream"() -> (w533:refnum<k24>)
            n337 = case shown="真" w532 {
              tunnel: w533 -> [_ w549]
              tunnel: w531 -> [_ w545]
              tunnel: w530 -> [w538 w548]
              tunnel: [w538 w544] -> w529
              tunnel: w528 -> [_ w542]
              frame False {
              }
              frame True {
                n338 = call <vilib>:"Acquire Semaphore.vi"("semaphore"=w542) -> ("semaphore out"=w541:T2)  [unwired: 4 in, 2 out]
                n339 = flat-sequence {
                  tunnel: w549 -> [w551]
                  tunnel: w548 -> [w553]
                  tunnel: [w553] -> w547
                  tunnel: [w552] -> w546
                  tunnel: w545 -> [w552]
                  tunnel: [w551] -> w543
                  tunnel: w541 -> [w550]
                  tunnel: [w550] -> w540
                  tunnel: [w562] -> w544
                  tunnel: w547 -> [w562]
                  tunnel: w546 -> [w561]
                  tunnel: w543 -> [w557]
                  tunnel: [w554] -> w539
                  tunnel: w540 -> [w554]
                  frame #0 {
                    n340 = call "StopGrab.vi"("IGxStream"=w551, "IGxDevice"=w553) -> ()  [unwired: 1 in, 1 out]
                  }
                  frame #1 {
                    n341 = local read "采集回调"() -> (w559:refnum<k27>)
                    n342 = Flush Event Queue(0:w561) -> (11:w560:errorcluster)  [unwired: 5 in, 2 out]
                    n343 = Unregister For Events(event registration refnum=w559, error in=w560) -> (error out=w556:errorcluster)
                    n344 = local write "采集状态"(FALSE) -> ()
                    n345 = call "CloseStream.vi"("error in (no error)"=w556) -> ("error out"=w558:errorcluster)  [unwired: 1 in]
                    n346 = Close Reference(reference=w557, error in (no error)=w558) -> ()  [unwired: 1 out]
                  }
                }
                n347 = call <vilib>:"Release Semaphore.vi"("semaphore"=w539) -> ()  [unwired: 5 in, 2 out]
              }
            }
            n348 = local read "设备状态"() -> (w534:bool)
            n349 = case shown="真" w534 {
              tunnel: w529 -> [_ w535]
              frame False {
              }
              frame True {
                n350 = call "CloseDevice.vi"("IGxDevice"=w535) -> ("error out"=w537:errorcluster)  [unwired: 1 in]
                n351 = local write "设备状态"(FALSE) -> ()
                n352 = Close Reference(reference=w535, error in (no error)=w537) -> ()  [unwired: 1 out]
              }
            }
          }
          frame #1 {
            n353 = local write "是否退出"(TRUE) -> ()
            n354 = Generate User Event(user event=w564, event data cluster="Quit") -> ()  [unwired: 2 in, 2 out]
          }
        }
      }
      event Panel Close? {
        n355 = event-data() -> ()  [unwired: 1 in, 4 out]
        n356 = flat-sequence {
          tunnel: w568 -> [w571]
          tunnel: w566 -> [w570]
          tunnel: w567 -> [w605]
          frame #0 {
            n357 = local read "采集状态"() -> (w574:bool)
            n358 = local read "IGxDevice"() -> (w573:refnum<k24>)
            n359 = local read "IGxStream"() -> (w575:refnum<k24>)
            n360 = case shown="真" w574 {
              tunnel: w575 -> [_ w591]
              tunnel: w571 -> [_ w587]
              tunnel: w573 -> [w580 w590]
              tunnel: [w580 w586] -> w572
              tunnel: w570 -> [_ w584]
              frame False {
              }
              frame True {
                n361 = call <vilib>:"Acquire Semaphore.vi"("semaphore"=w584) -> ("semaphore out"=w583:T2)  [unwired: 4 in, 2 out]
                n362 = flat-sequence {
                  tunnel: w591 -> [w593]
                  tunnel: w590 -> [w595]
                  tunnel: [w595] -> w589
                  tunnel: [w594] -> w588
                  tunnel: w587 -> [w594]
                  tunnel: [w593] -> w585
                  tunnel: w583 -> [w592]
                  tunnel: [w592] -> w582
                  tunnel: [w604] -> w586
                  tunnel: w589 -> [w604]
                  tunnel: w588 -> [w603]
                  tunnel: w585 -> [w599]
                  tunnel: [w596] -> w581
                  tunnel: w582 -> [w596]
                  frame #0 {
                    n363 = call "StopGrab.vi"("IGxStream"=w593, "IGxDevice"=w595) -> ()  [unwired: 1 in, 1 out]
                  }
                  frame #1 {
                    n364 = local read "采集回调"() -> (w601:refnum<k27>)
                    n365 = Flush Event Queue(0:w603) -> (11:w602:errorcluster)  [unwired: 5 in, 2 out]
                    n366 = Unregister For Events(event registration refnum=w601, error in=w602) -> (error out=w598:errorcluster)
                    n367 = local write "采集状态"(FALSE) -> ()
                    n368 = call "CloseStream.vi"("error in (no error)"=w598) -> ("error out"=w600:errorcluster)  [unwired: 1 in]
                    n369 = Close Reference(reference=w599, error in (no error)=w600) -> ()  [unwired: 1 out]
                  }
                }
                n370 = call <vilib>:"Release Semaphore.vi"("semaphore"=w581) -> ()  [unwired: 5 in, 2 out]
              }
            }
            n371 = local read "设备状态"() -> (w576:bool)
            n372 = case shown="真" w576 {
              tunnel: w572 -> [_ w577]
              frame False {
              }
              frame True {
                n373 = call "CloseDevice.vi"("IGxDevice"=w577) -> ("error out"=w579:errorcluster)  [unwired: 1 in]
                n374 = local write "设备状态"(FALSE) -> ()
                n375 = Close Reference(reference=w577, error in (no error)=w579) -> ()  [unwired: 1 out]
              }
            }
          }
          frame #1 {
            n376 = local write "是否退出"(TRUE) -> ()
            n377 = Generate User Event(user event=w605, event data cluster="Quit") -> ()  [unwired: 2 in, 2 out]
          }
        }
        n378 = event-data() -> ()  [unwired: 2 in, 1 out]
      }
    }
    "error out" <- w355
    n379 = call <vilib>:"Simple Error Handler.vi"("error in (no error)"=w355) -> ()  [unwired: 4 in, 5 out]
  }
  n380 = Stop(stop? (T)=w4) -> ()
